vi "Read View Settings.vi"(0 "Controller in":refnum<class "Controller.lvclass">, 1 "View Name":string, 5 "error in (no error)":errorcluster) -> (14 "Controller out":refnum<class "Controller.lvclass">, 19 "error out":errorcluster)   [LabVIEW 2023, in "MVC Actors.lvlib" / "Controller.lvclass"]
doc: "Allows the child controller to get the behavior of a View actor specified in the <b>View Name</b> by registering to the user defined event whose reference is accessible by the <b>View Settings Event Ref</b> property that will deliver the following settings\n\n<b>Exclude From Broadcast</b>: message originating form another View will not be broadcasted to the View being cosidered\n<b>Paused</b>: the View will not send events and will not receive them anymore\n<b>Receive only</b>: The View will receive events but not send any"
uses:
  Controller.lvclass
  Controller.lvclass/Controller.ctl
  View Details.ctl
  <vilib>/ActorFramework/Message Enqueuer/Message Enqueuer.lvclass
  View Settings.ctl
panel:
  out "View Not Found":bool
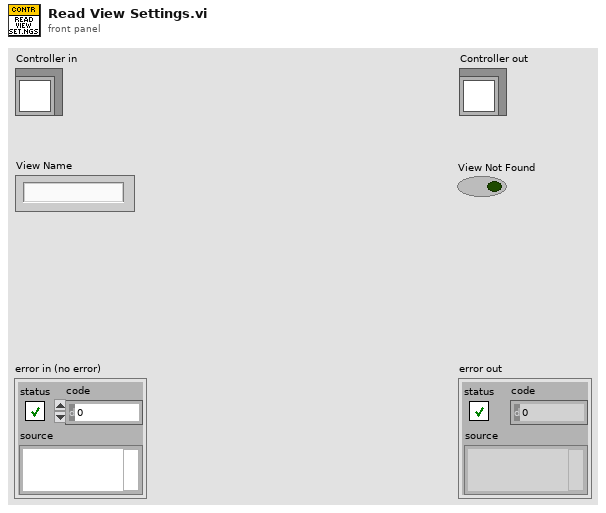
[diagram p1: front panel]
types:
  T1 = typedef "MVC Actors.lvlib/Controller.lvclass/View Settings Event Ref.ctl" = refnum<user-event>
  T2 = typedef "MVC Actors.lvlib/Controller.lvclass/View Settings.ctl" = cluster{"Exclude From Broadcast":bool, "Receive Only":bool, "Paused":bool}
  T3 = typedef "MVC Actors.lvlib/Controller.lvclass/View Details.ctl" = cluster{"Exclude From Broadcast":bool, "Receive Only":bool, "Paused":bool, "View Enqueuer":refnum<class "Message Enqueuer.lvclass">}
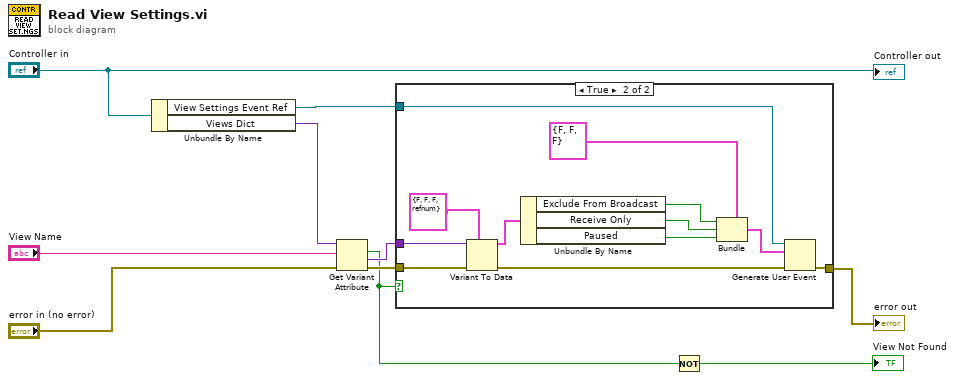
[diagram p0: block diagram]
diagram:
  n1 = Unbundle By Name("Controller in") -> ("View Settings Event Ref"=w1:T1, "Views Dict"=w8:variant)
  n2 = Get Variant Attribute(Variant=w8, name="View Name", error in="error in (no error)") -> (found=w3:bool, value=w9:variant, error out=w10:errorcluster)  [unwired: 1 in, 1 out]
  n3 = case shown="True" w3 {
    tunnel: w9 -> [_ w22]
    tunnel: w10 -> [w11 w23]
    tunnel: [w11 w14] -> w4
    tunnel: w1 -> [_ w13]
    frame False {
    }
    frame True {
      n4 = Variant To Data(error in=w23, type=T3 {"Exclude From Broadcast"=FALSE, "Receive Only"=FALSE, "Paused"=FALSE, "View Enqueuer"=refnum} ("Message Enqueuer"), Variant=w22) -> (data=w20:T3, error out=w15:errorcluster)
      n5 = Unbundle By Name(w20) -> ("Exclude From Broadcast"=w18:bool, "Receive Only"=w17:bool, "Paused"=w16:bool)
      n6 = Bundle(cluster=T2 {"Exclude From Broadcast"=FALSE, "Receive Only"=FALSE, "Paused"=FALSE} ("Sink Settings"), "Exclude From Broadcast"=w18, "Receive Only"=w17, "Paused"=w16) -> (w12:T2)
      n7 = Generate User Event(user event=w13, event data cluster=w12, error in=w15) -> (error out=w14:errorcluster)  [unwired: 1 in, 1 out]
    }
  }
  "error out" <- w4
  n8 = Not(x=w3) -> (.not. x?=→"View Not Found":bool)
  "Controller out" <- "Controller in"
